vi "example test.vi"() -> ()   [LabVIEW 2013, in "UI reference module tests.lvlib"]
uses:
  UI reference module tests.lvlib
  module/execution/UI Reference runtime.lvclass
  module/configuration/UI Reference configuration.lvclass
  module/configuration/UI Reference configuration.lvclass/UI Reference configuration.ctl
  <vilib>/NI/Tag Bus/dictionary/data dictionary.lvclass/data dictionary.ctl
  <vilib>/NI/Tag Bus/dictionary/lookup polymorphs/locate double.vi
  <vilib>/NI/Tag Bus/dictionary/lookup polymorphs/locate Boolean.vi
  <vilib>/NI/Tag Bus/dictionary/lookup polymorphs/locate String.vi
  <vilib>/NI/Tag Bus/table/data polymorphs/read one/read Double.vi
  <vilib>/NI/Tag Bus/table/data polymorphs/read one/read Boolean.vi
  <vilib>/NI/Tag Bus/table/data polymorphs/read one/read String.vi
  <vilib>/NI/Tag Bus/table/data polymorphs/write one/write Double.vi
  <vilib>/NI/Tag Bus/table/data polymorphs/write one/write Boolean.vi
  <vilib>/NI/Tag Bus/table/data polymorphs/write one/write String.vi
  module/configuration/Write VI Refnum.vi
  <vilib>/NI/Tag Bus/dictionary/search/find data index.vi
  <vilib>/NI/Tag Bus/dictionary/search/search string list.vi
  <vilib>/NI/Tag Bus/dictionary/tag not found.vi
  <vilib>/NI/Tag Bus/dictionary/data dictionary.lvclass
  <vilib>/NI/Tag Bus/table/data table.lvlib
panel:
  out "exec settings":errorcluster
  in  "Stop wkaround":errorcluster
  out "String out":string
  in  "String in":string
  out "bool out":bool
  in  "bool in":bool
  out "dbl out":dbl
  in  "dbl in":dbl
  out "final error":errorcluster
  out "init error":errorcluster
  out "serialization problem":errorcluster
  out "invalid configuration":errorcluster
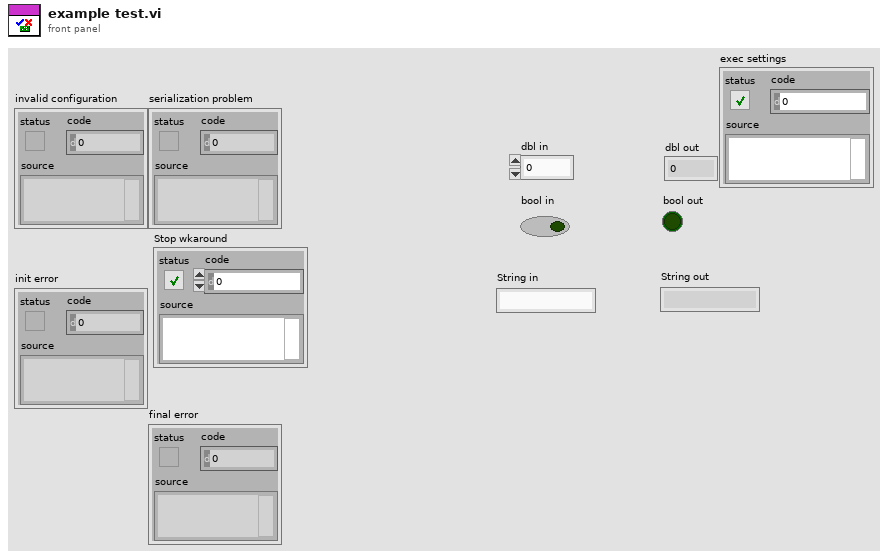
[diagram p1: front panel]
types:
  T1 = typedef "TBM channel.lvclass/data tables.ctl" = cluster{"input data":T2, "processing parameter":T2, "processing result":T2, "output data":T2}
  T2 = typedef "tag bus.lvlib/dictionary table pair.ctl" = cluster{"data dictionary":refnum<class "data dictionary.lvclass">, "data table":T3}
  T3 = typedef "tag bus.lvlib/data table.lvlib/data table.ctl" = cluster{"Double":dbl[], "Single":sgl[], "I64":i64[], "I32":i32[], "I16":i16[], "I8":i8[], "U64":u64[], "U32":u32[], "U16":u16[], "U8":u8[], "Boolean":bool[], "String":string[], "Array of Double":cluster{"DBL Array":dbl[]}[], "Array of Single":cluster{"SGL Array":sgl[]}[], "Array of I64":cluster{"I64 Array":i64[]}[], "Array of I32":cluster{"I32 Array":i32[]}[], "Array of I16":cluster{"I16 Array":i16[]}[], "Array of I8":cluster{"I8 Array":i8[]}[], "Array of U64":cluster{"U64 Array":u64[]}[], "Array of U32":cluster{"U32 Array":u32[]}[], "Array of U16":cluster{"U16 Array":u16[]}[], "Array of U8":cluster{"U8 Array":u8[]}[], "Array of Boolean":cluster{"Boolean Array":bool[]}[], "Array of String":cluster{"String Array":string[]}[]}
  T4 = typedef "TBM module execution interface.lvclass/execution settings.ctl" = cluster{"reads inputs":bool, "processes data":bool, "writes outputs":bool}
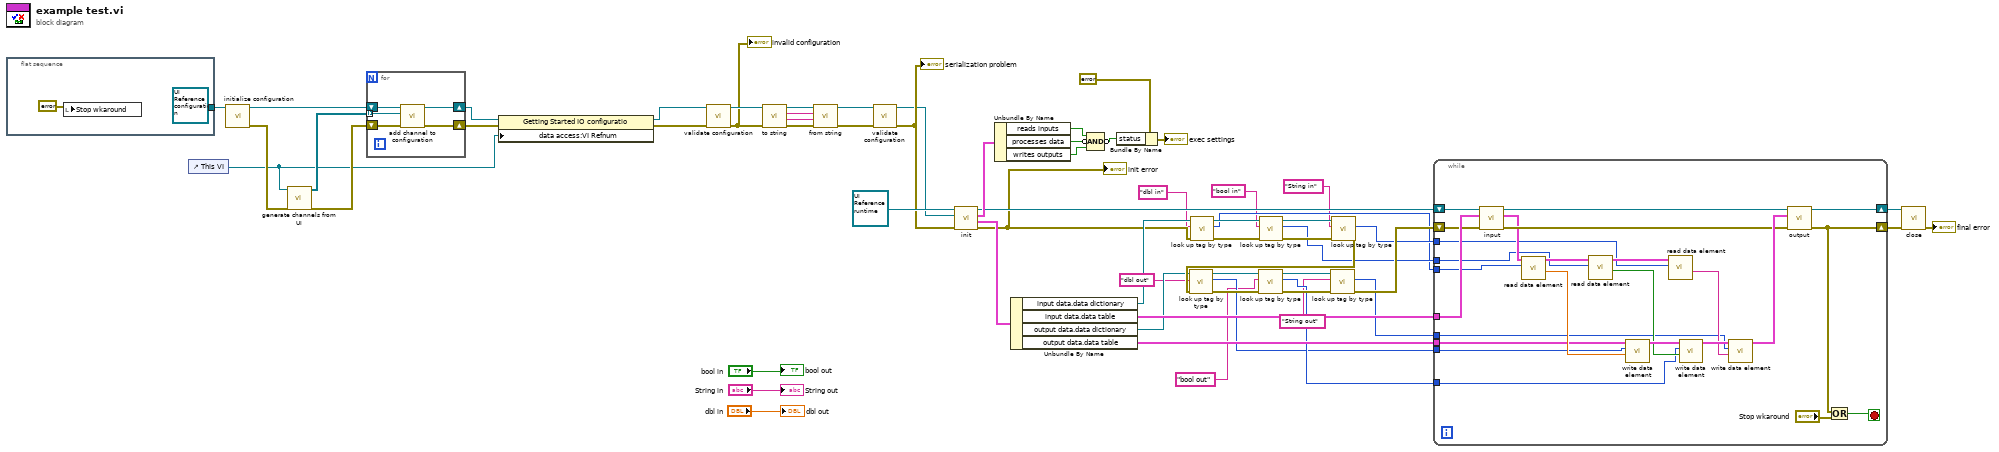
[diagram p0: block diagram]
diagram:
  n1 = flat-sequence {
    tunnel: [refnum<class "UI Reference configuration.lvclass"> refnum ("tag bus configurable plugin module configuration")] -> w43
    frame #0 {
      n2 = local write "Stop wkaround"(errorcluster {"status"=FALSE, "code"=0, "source"=""} ("Stop wkaround")) -> ()
    }
  }
  n3 = control-ref of="This VI"() -> (w34:refnum<vi>)
  n4 = call-dynamic "initialize configuration.vi"("configuration in"=w43) -> ("error out"=w41:errorcluster, "configuration out"=w38:refnum<class "UI Reference configuration.lvclass">)  [unwired: 8 in, 1 out]
  n5 = call "generate channels from UI.vi"("error in"=w41, "VI Refnum"=w34) -> ("error out"=w40:errorcluster, "channels"=w39:refnum<class "TBM channel.lvclass">[])  [unwired: 8 in]
  n6 = for {
    shift-right: [w70] -> w36
    shift-left: w38 -> [w68]
    shift-right: [w69] -> w42
    shift-left: w40 -> [w67]
    tunnel: w39 -> [w66] mode=indexing
    n7 = call "add channel to configuration.vi"("error in"=w67, "channel"=w66, "Getting Started IO configuration in"=w68) -> ("error out"=w69:errorcluster, "Getting Started IO configuration out"=w70:refnum<class "UI Reference configuration.lvclass">)  [unwired: 7 in]
  }
  n8 = property class="Getting Started IO configuratio"(reference=w36, error in=w42, "data access:VI Refnum"=w34) -> (reference out=w35:refnum<class "UI Reference configuration.lvclass">, error out=w37:errorcluster)
  n9 = call-dynamic "validate configuration.vi"("error in"=w37, "Getting Started IO configuration in"=w35) -> ("error out"=w62:errorcluster, "Getting Started IO configuration out"=w63:refnum<class "UI Reference configuration.lvclass">)  [unwired: 8 in]
  "invalid configuration" <- w62
  n10 = call-dynamic "to string.vi"("error in"=w62, "Getting Started IO configuration in"=w63) -> ("error out"=w58:errorcluster, "data"=w59:string, "version"=w60:string, "Getting Started IO configuration out"=w61:refnum<class "UI Reference configuration.lvclass">)  [unwired: 6 in]
  n11 = call-dynamic "from string.vi"("error in"=w58, "data"=w59, "version"=w60, "Getting Started IO configuration in"=w61) -> ("error out"=w56:errorcluster, "Getting Started IO configuration out"=w57:refnum<class "UI Reference configuration.lvclass">)  [unwired: 6 in]
  n12 = call-dynamic "validate configuration.vi"("error in"=w56, "Getting Started IO configuration in"=w57) -> ("error out"=w54:errorcluster, "Getting Started IO configuration out"=w53:refnum<class "UI Reference configuration.lvclass">)  [unwired: 8 in]
  "serialization problem" <- w54
  n13 = call-dynamic "init.vi"("error in"=w54, "TBM module configuration in"=w53, "Getting Started IO runtime in"=refnum<class "UI Reference runtime.lvclass"> refnum ("tag bus configurable plugin module")) -> ("error out"=w20:errorcluster, "data allocations"=w48:T1, "execution settings"=w52:T4, "Getting Started IO runtime out"=w47:refnum<class "UI Reference runtime.lvclass">)  [unwired: 5 in]
  "init error" <- w20
  n14 = Unbundle By Name(w52) -> ("reads inputs"=w49:bool, "processes data"=w51:bool, "writes outputs"=w50:bool)
  n15 = Unbundle By Name(w48) -> ("input data.data dictionary"=w21:refnum<class "data dictionary.lvclass">, "input data.data table"=w32:T3, "output data.data dictionary"=w24:refnum<class "data dictionary.lvclass">, "output data.data table"=w33:T3)
  n16 = Compound Arithmetic op=AND(w49, invert w51, w50) -> (invert w5:bool)
  n17 = Bundle By Name(cluster=errorcluster {"status"=FALSE, "code"=0, "source"=""} ("error out"), "status"=w5) -> (→"exec settings":errorcluster)
  n18 = call-poly <vilib>:"look up tag by type.vi"("error in"=w20, "name"="dbl in", "data dictionary in"=w21) -> ("error out"=w30:errorcluster, "index"=w16:i32, "data dictionary out"=w31:refnum<class "data dictionary.lvclass">)  [unwired: 6 in]
  n19 = call-poly <vilib>:"look up tag by type.vi"("error in"=w30, "name"="bool in", "data dictionary in"=w31) -> ("error out"=w28:errorcluster, "index"=w17:i32, "data dictionary out"=w29:refnum<class "data dictionary.lvclass">)  [unwired: 6 in]
  n20 = call-poly <vilib>:"look up tag by type.vi"("error in"=w28, "name"="String in", "data dictionary in"=w29) -> ("error out"=w25:errorcluster, "index"=w18:i32)  [unwired: 6 in, 1 out]
  n21 = call-poly <vilib>:"look up tag by type.vi"("error in"=w25, "name"="dbl out", "data dictionary in"=w24) -> ("error out"=w26:errorcluster, "index"=w13:i32, "data dictionary out"=w23:refnum<class "data dictionary.lvclass">)  [unwired: 6 in]
  n22 = call-poly <vilib>:"look up tag by type.vi"("error in"=w26, "name"="bool out", "data dictionary in"=w23) -> ("error out"=w27:errorcluster, "index"=w14:i32, "data dictionary out"=w22:refnum<class "data dictionary.lvclass">)  [unwired: 6 in]
  n23 = call-poly <vilib>:"look up tag by type.vi"("error in"=w27, "name"="String out", "data dictionary in"=w22) -> ("error out"=w19:errorcluster, "index"=w15:i32)  [unwired: 6 in, 1 out]
  n24 = while {
    tunnel: w33 -> [w83]
    tunnel: w32 -> [w82]
    shift-right: [w79] -> w45
    shift-left: w19 -> [w81]
    shift-right: [w92] -> w46
    shift-left: w47 -> [w95]
    tunnel: w18 -> [w76]
    tunnel: w17 -> [w75]
    tunnel: w16 -> [w74]
    tunnel: w15 -> [w73]
    tunnel: w14 -> [w72]
    tunnel: w13 -> [w71]
    stop <- w77 stop-if-true
    n25 = call-dynamic "input.vi"("error in"=w81, "data table in"=w82, "Getting Started IO runtime in"=w95) -> ("error out"=w91:errorcluster, "data table out"=w80:T3, "Getting Started IO runtime out"=w94:refnum<class "UI Reference runtime.lvclass">)  [unwired: 6 in]
    n26 = call-poly <vilib>:"read data element.vi"("index"=w74, "data table in"=w80) -> ("value"=w84:dbl, "data table out"=w88:T3)  [unwired: 8 in]
    n27 = call-poly <vilib>:"read data element.vi"("index"=w75, "data table in"=w88) -> ("value"=w85:bool, "data table out"=w87:T3)  [unwired: 8 in]
    n28 = call-poly <vilib>:"write data element.vi"("value"=w84, "index"=w71, "data table in"=w83) -> ("data table out"=w89:T3)  [unwired: 8 in]
    n29 = call-poly <vilib>:"read data element.vi"("index"=w76, "data table in"=w87) -> ("value"=w86:string)  [unwired: 8 in, 1 out]
    n30 = call-poly <vilib>:"write data element.vi"("value"=w85, "index"=w72, "data table in"=w89) -> ("data table out"=w90:T3)  [unwired: 8 in]
    n31 = call-poly <vilib>:"write data element.vi"("value"=w86, "index"=w73, "data table in"=w90) -> ("data table out"=w93:T3)  [unwired: 8 in]
    n32 = call-dynamic "output.vi"("error in"=w91, "data table in"=w93, "Getting Started IO runtime in"=w94) -> ("error out"=w79:errorcluster, "Getting Started IO runtime out"=w92:refnum<class "UI Reference runtime.lvclass">)  [unwired: 6 in, 1 out]
    n33 = Or(x=w79, y="Stop wkaround") -> (x .or. y?=w77:bool)
  }
  n34 = call-dynamic "close.vi"("error in"=w45, "Getting Started IO runtime in"=w46) -> ("error out"=→"final error":errorcluster)  [unwired: 9 in]
  "dbl out" <- "dbl in"
  "bool out" <- "bool in"
  "String out" <- "String in"
